vi "Select Key Files.vi"(8 "Error In":errorcluster, 11 "Key Files In":cluster{"Private":path, "Public":path}={"Private"=path "", "Public"=path ""}) -> (0 "Error Out":errorcluster, 3 "Key Files Out":cluster{"Private":path, "Public":path})   [LabVIEW 2017, in "Tests.lvlib"]
uses:
  Tests.lvlib
  SSH Key Types.ctl
  <vilib>/Utility/file.llb/Is Path and Not Empty.vi
  <vilib>/Utility/sysdir.llb/Get System Directory.vi
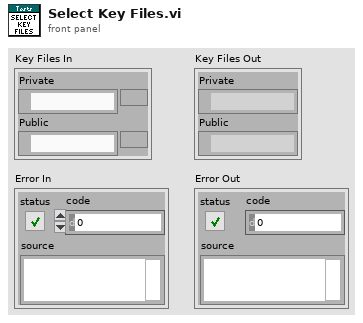
[diagram p1: front panel]
types:
  T1 = typedef "Tests.lvlib/SSH Key Types.ctl" = enum16{"Private", "Public"}
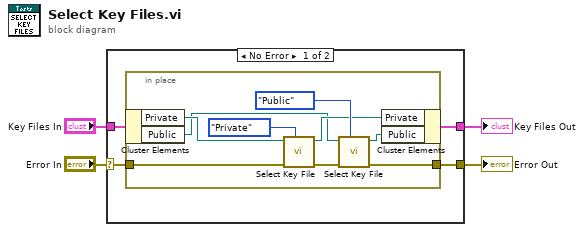
[diagram p0: block diagram]
diagram:
  n1 = case shown="No Error" "Error In" {
    selector: "Error In" -> [w5 w18]
    tunnel: [w8 w18] -> w4
    tunnel: "Key Files In" -> [w7 w19]
    tunnel: [w6 w19] -> w2
    frame No Error {
      n2 = in-place {
        in-place-border: [w16] -> w8
        in-place-border: w5 -> [w13]
        n3 = in-place-cluster #1(w7) -> ("Private"=w12:path, "Public"=w10:path)
        n4 = call "Select Key File.vi"("Key Type"=SSH_Key_Types."Private", "Error In"=w13, "Key File In"=w12) -> ("Error Out"=w15:errorcluster, "Key File Out"=w11:path)  [unwired: 7 in]
        n5 = call "Select Key File.vi"("Key Type"=SSH_Key_Types."Public", "Error In"=w15, "Key File In"=w10) -> ("Error Out"=w16:errorcluster, "Key File Out"=w9:path)  [unwired: 7 in]
        n6 = in-place-cluster #1("Private"=w11, "Public"=w9) -> (w6:cluster{"Private":path, "Public":path})
      }
    }
    frame Error {
    }
  }
  "Error Out" <- w4
  "Key Files Out" <- w2
